vi "CompileParseMWPulse.vi"(1 "Pulse List In":T2[](array[typedef])) -> (0 "Pulse seq out":T1(array[cluster]))   [LabVIEW 2019]
uses:
  SinglePulse.ctl
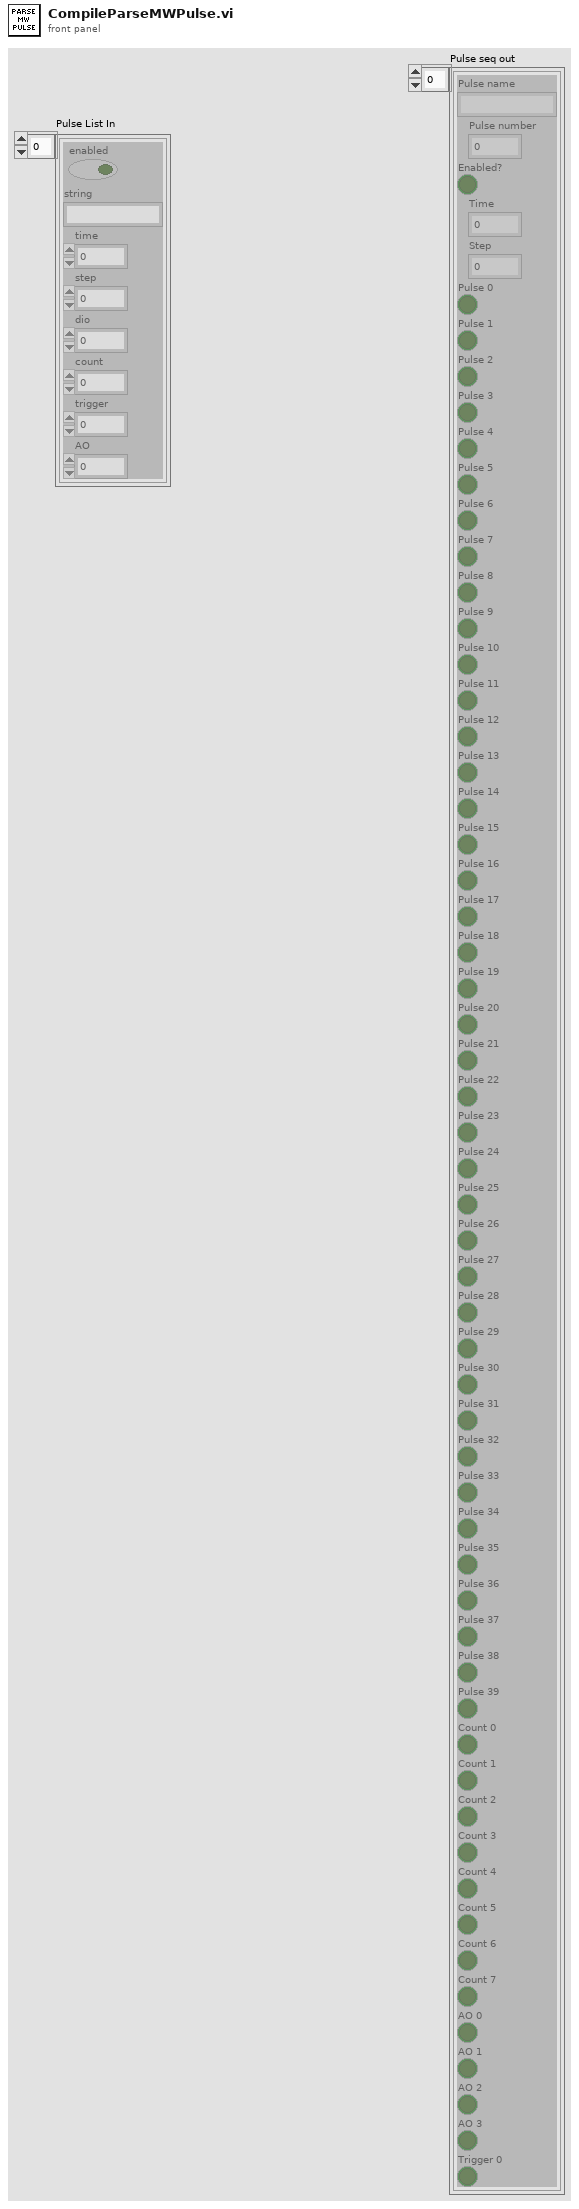
[diagram p1: front panel]
types:
  T1 = cluster{"Pulse name":string, "Pulse number":i32, "Enabled?":bool, "Time":dbl, "Step":dbl, "Pulse 0":bool, "Pulse 1":bool, "Pulse 2":bool, "Pulse 3":bool, "Pulse 4":bool, "Pulse 5":bool, "Pulse 6":bool, "Pulse 7":bool, "Pulse 8":bool, "Pulse 9":bool, "Pulse 10":bool, "Pulse 11":bool, "Pulse 12":bool, "Pulse 13":bool, "Pulse 14":bool, "Pulse 15":bool, "Pulse 16":bool, "Pulse 17":bool, "Pulse 18":bool, "Pulse 19":bool, "Pulse 20":bool, "Pulse 21":bool, "Pulse 22":bool, "Pulse 23":bool, "Pulse 24":bool, "Pulse 25":bool, "Pulse 26":bool, "Pulse 27":bool, "Pulse 28":bool, "Pulse 29":bool, "Pulse 30":bool, "Pulse 31":bool, "Pulse 32":bool, "Pulse 33":bool, "Pulse 34":bool, "Pulse 35":bool, "Pulse 36":bool, "Pulse 37":bool, "Pulse 38":bool, "Pulse 39":bool, "Count 0":bool, "Count 1":bool, "Count 2":bool, "Count 3":bool, "Count 4":bool, "Count 5":bool, "Count 6":bool, "Count 7":bool, "AO 0":bool, "AO 1":bool, "AO 2":bool, "AO 3":bool, "Trigger 0":bool}[]
  T2 = typedef "SinglePulse.ctl" = cluster{"enabled":bool, "string":string, "time":dbl, "step":dbl, "dio":dbl, "count":dbl, "trigger":dbl, "AO":dbl}
  T3 = cluster{"Pulse name":string, "Pulse number":i32, "Enabled?":bool, "Time":dbl, "Step":dbl, "Pulse 0":bool, "Pulse 1":bool, "Pulse 2":bool, "Pulse 3":bool, "Pulse 4":bool, "Pulse 5":bool, "Pulse 6":bool, "Pulse 7":bool, "Pulse 8":bool, "Pulse 9":bool, "Pulse 10":bool, "Pulse 11":bool, "Pulse 12":bool, "Pulse 13":bool, "Pulse 14":bool, "Pulse 15":bool, "Pulse 16":bool, "Pulse 17":bool, "Pulse 18":bool, "Pulse 19":bool, "Pulse 20":bool, "Pulse 21":bool, "Pulse 22":bool, "Pulse 23":bool, "Pulse 24":bool, "Pulse 25":bool, "Pulse 26":bool, "Pulse 27":bool, "Pulse 28":bool, "Pulse 29":bool, "Pulse 30":bool, "Pulse 31":bool, "Pulse 32":bool, "Pulse 33":bool, "Pulse 34":bool, "Pulse 35":bool, "Pulse 36":bool, "Pulse 37":bool, "Pulse 38":bool, "Pulse 39":bool, "Count 0":bool, "Count 1":bool, "Count 2":bool, "Count 3":bool, "Count 4":bool, "Count 5":bool, "Count 6":bool, "Count 7":bool, "AO 0":bool, "AO 1":bool, "AO 2":bool, "AO 3":bool, "Trigger 0":bool}
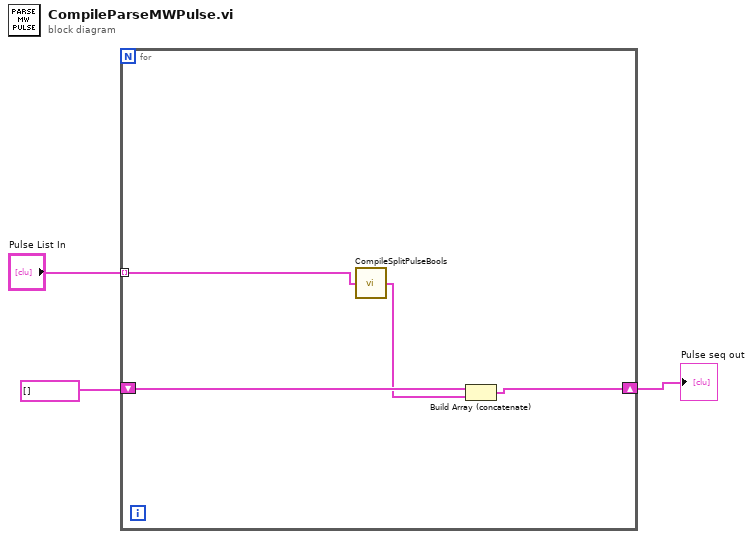
[diagram p0: block diagram]
diagram:
  n1 = for {
    tunnel: "Pulse List In" -> [w4] mode=indexing
    shift-right: [w6] -> w1
    shift-left: T1 [] -> [w7]
    n2 = call "CompileSplitPulseBools.vi"("Singe pulse"=w4) -> ("Bool pulse out"=w5:T3)
    n3 = Build Array (concatenate)(w7, w5) -> (w6:T1)
  }
  "Pulse seq out" <- w1
